vi "Sequence Array Formatting.vi"(0 "Sequence Array":string[](array[string])=["Connect Test", "PSU Test", "LED Test", "Fake test", "Fake test", "Fake test", "Fake test", "Fake test", "Fake test", "Fake test", "Fake test"], 11 "error in":errorcluster) -> (4 "Formatted Sequence":string, 15 "error out":errorcluster)   [LabVIEW 2024]
uses:
  <userlib>/_OpenG.lib/string/string.llb/openg_string.lvlib
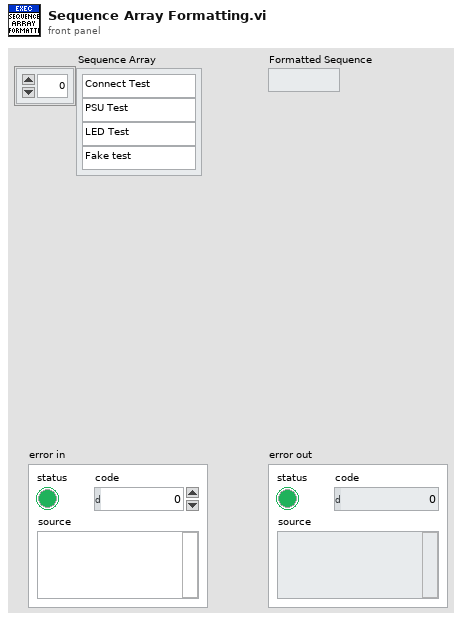
[diagram p1: front panel]
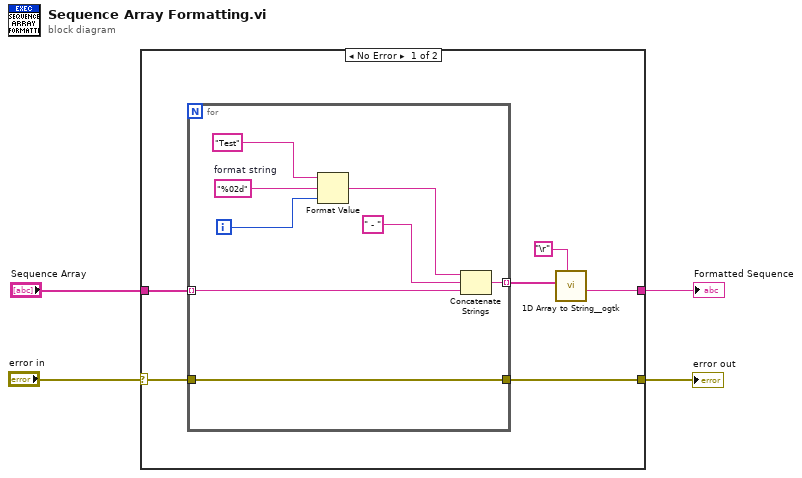
[diagram p0: block diagram]
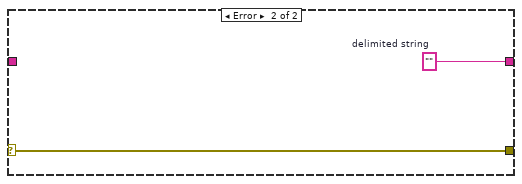
[diagram p2: hidden frame]
diagram:
  n1 = case shown="No Error" "error in" {
    selector: "error in" -> [w9 w19]
    tunnel: "Sequence Array" -> [w10 _]
    tunnel: [w8 w19] -> w2
    tunnel: [w5 w20] -> w1
    frame No Error {
      n2 = for {
        tunnel: w10 -> [w17] mode=indexing
        tunnel: [w18] -> w6 mode=indexing
        tunnel: w9 -> [w11]
        tunnel: [w11] -> w8
        i -> [w16]
        w15 = "%02d"  # format string
        n3 = Format Value(string ("")="Test", format string=w15, value (0)=w16) -> (output string=w13:string)
        n4 = Concatenate Strings(w13, " - ", w17) -> (w18:string)
      }
      n5 = call <userlib>:"1D Array to String__ogtk.vi"("delimiter (Tab)"="\r", "Array of Strings"=w6) -> ("delimited string"=w5:string)  [unwired: 9 in]
    }
    frame Error {
      w20 = ""  # delimited string
    }
  }
  "error out" <- w2
  "Formatted Sequence" <- w1
